vi "Colour to CMYK.vi"(0 "Colour":u32(colorbox), 11 "error in (no error)":errorcluster) -> (3 "Resolved Colour":u32 format="%.0x", 4 "Cyan(%)":dbl format="%#_13g", 6 "Magenta(%)":dbl format="%#_13g", 8 "Yellow(%)":dbl format="%#_13g", 10 "Key/Black(%)":dbl format="%#.2g", 15 "error out":errorcluster)   [LabVIEW 2018, in "Colour Lab.lvlib"]
uses:
  Colour Lab.lvlib
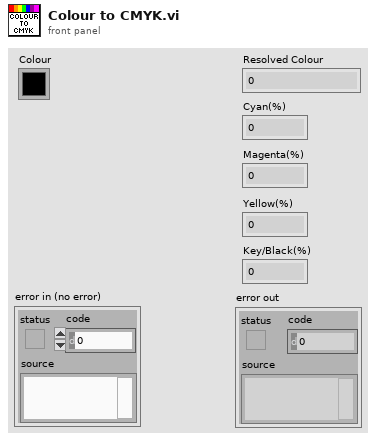
[diagram p1: front panel]
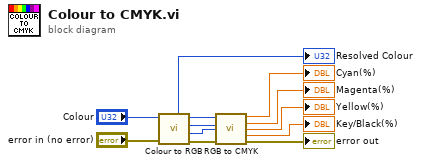
[diagram p0: block diagram]
diagram:
  n1 = call "Colour to RGB.vi"("error in (no error)"="error in (no error)", "Colour"="Colour") -> ("error out"=w12:errorcluster, "Blue"=w11:u8, "Green"=w3:u8, "Red"=w10:u8, "Resolved Colour"=→"Resolved Colour":u32)  [unwired: 5 in]
  n2 = call "RGB to CMYK.vi"("Red"=w10, "Green"=w3, "Blue"=w11, "error in (no error)"=w12) -> ("Cyan(%)"=→"Cyan(%)":dbl, "Magenta(%)"=→"Magenta(%)":dbl, "Yellow(%)"=→"Yellow(%)":dbl, "Key/Black(%)"=→"Key/Black(%)":dbl, "error out"=→"error out":errorcluster)  [unwired: 7 in]
